vi "test-ElevatorSim-min-max.vi"() -> (3 "Test Passed":bool)   [LabVIEW 2019]
uses:
  <vilib>/Rock Robotics/WPI/ThirdParty/JAS_Junk/TrajLib/DCMOTOR.CTL
  <vilib>/Rock Robotics/WPI/ThirdParty/JAS_Junk/TrajLib/ELEVATOR_SIM.ctl
  <vilib>/Rock Robotics/WPI/ThirdParty/JAS_Junk/TrajLib/LINEAR_SYSTEM_SIM.ctl
  <vilib>/Rock Robotics/WPI/ThirdParty/JAS_Junk/TrajLib/LINEAR_SYSTEM.ctl
  <vilib>/Analysis/Matrix/Datatypes/RealMatrix.ctl
  <vilib>/Rock Robotics/WPI/ThirdParty/JAS_Junk/TrajLib/DCMotor_New.vi
  <vilib>/Rock Robotics/WPI/ThirdParty/JAS_Junk/TrajLib/Units_RotationsPerMinuteToRadiansPerSecond.vi
  <vilib>/Rock Robotics/WPI/ThirdParty/JAS_Junk/TrajLib/MatBuilder_Create.vi
  <vilib>/Rock Robotics/WPI/ThirdParty/JAS_Junk/TrajLib/MatBuilder_Fill.vi
  <vilib>/Rock Robotics/WPI/ThirdParty/JAS_Junk/TrajLib/MatrixHelper_Zero.vi
  <vilib>/Rock Robotics/WPI/ThirdParty/JAS_Junk/TrajLib/LinearSystem_New.vi
  <vilib>/Rock Robotics/WPI/ThirdParty/JAS_Junk/TrajLib/Trajectory_Library.lvlib
  <vilib>/Analysis/Matrix/NI_Matrix.lvlib
panel:
  in  "Tab Control":enum32{"Page 2", "Page 6", "Page 7"}(tab)
  out "Elevator Motor":T1 {"Jr_KgM2" format="%13.5p"; "L_H" format="%13.5p"; "Kt_NMPerAmp" format="%13.5p"; "KvINV_RadPerSecPerVolt" format="%13.5p"; "R_Ohms" format="%13.5p"; "FreeSpeed_RadPerSec" format="%13.5p"; "FreeCurrent_Amps" format="%13.5p"; "StallCurrent_Amps" format="%13.5p"; "StallTorque_NM" format="%13.5p"; "nominalVoltage_Volts" format="%13.5p"}
  out "Elevator Simulaation":T2 {"GearBox"."Jr_KgM2" format="%13.5p"; "GearBox"."L_H" format="%13.5p"; "GearBox"."Kt_NMPerAmp" format="%13.5p"; "GearBox"."KvINV_RadPerSecPerVolt" format="%13.5p"; "GearBox"."R_Ohms" format="%13.5p"; "GearBox"."FreeSpeed_RadPerSec" format="%13.5p"; "GearBox"."FreeCurrent_Amps" format="%13.5p"; "GearBox"."StallCurrent_Amps" format="%13.5p"; "GearBox"."StallTorque_NM" format="%13.5p"; "GearBox"."nominalVoltage_Volts" format="%13.5p"}
  out "Velocity":cluster{"Voltage":dbl}(graph)
  out "PV Chart":cluster{dbl}(graph)
  out "At Top":bool
  out "At Bottom":bool
  out "PV Chart 2":cluster{dbl}(graph)
  out "At Bottom 2":bool
  out "At Top 2":bool
  out "Velocity 2":cluster{"Voltage":dbl}(graph)
  # "<States, 1>"
  # "<Outputs, 1>"
  # "<Inputs, 1>"
  # "<Outputs, 1>"
  # "<States,States>"
  # "<States,Inputs>"
  # "<Outputs,States>"
  # "<Outputs,Inputs>"
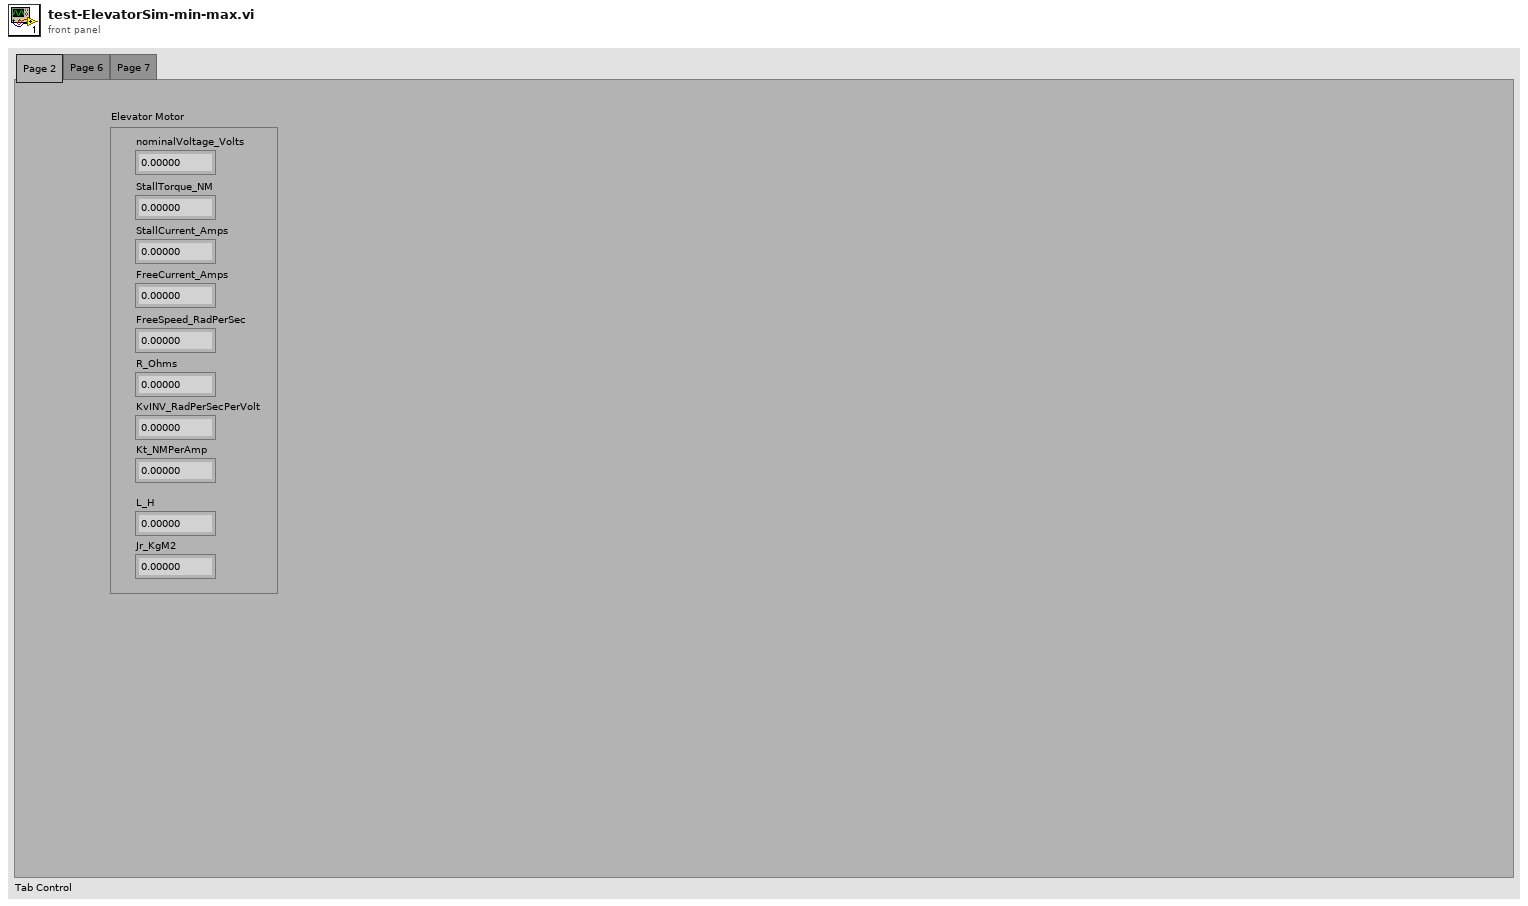
[diagram p1: front panel]
types:
  T1 = typedef "Trajectory_Library.lvlib/DCMOTOR.CTL" = cluster{"nominalVoltage_Volts":dbl, "StallTorque_NM":dbl, "StallCurrent_Amps":dbl, "FreeCurrent_Amps":dbl, "FreeSpeed_RadPerSec":dbl, "R_Ohms":dbl, "KvINV_RadPerSecPerVolt":dbl, "Kt_NMPerAmp":dbl, "L_H":dbl, "Jr_KgM2":dbl}
  T2 = typedef "Trajectory_Library.lvlib/ELEVATOR_SIM.ctl" = cluster{"LinearSystemSim":T3, "GearBox":T1, "Gearing":dbl, "DrumRadius_M":dbl, "MinHeight_M":dbl, "MaxHeight_M":dbl, "CarriageMass_Kg":dbl}
  T3 = typedef "Trajectory_Library.lvlib/LINEAR_SYSTEM_SIM.ctl" = cluster{"m_Plant":T4, "m_X":T5, "m_Y":T5, "m_U":T5, "MeasureStdDev":T5}
  T4 = typedef "Trajectory_Library.lvlib/LINEAR_SYSTEM.ctl" = cluster{"m_A":T5, "m_B":T5, "m_C":T5, "m_D":T5, "States":i32, "Inputs":i32, "Outputs":i32}
  T5 = typedef "NI_Matrix.lvlib/RealMatrix.ctl" = dbl[][]
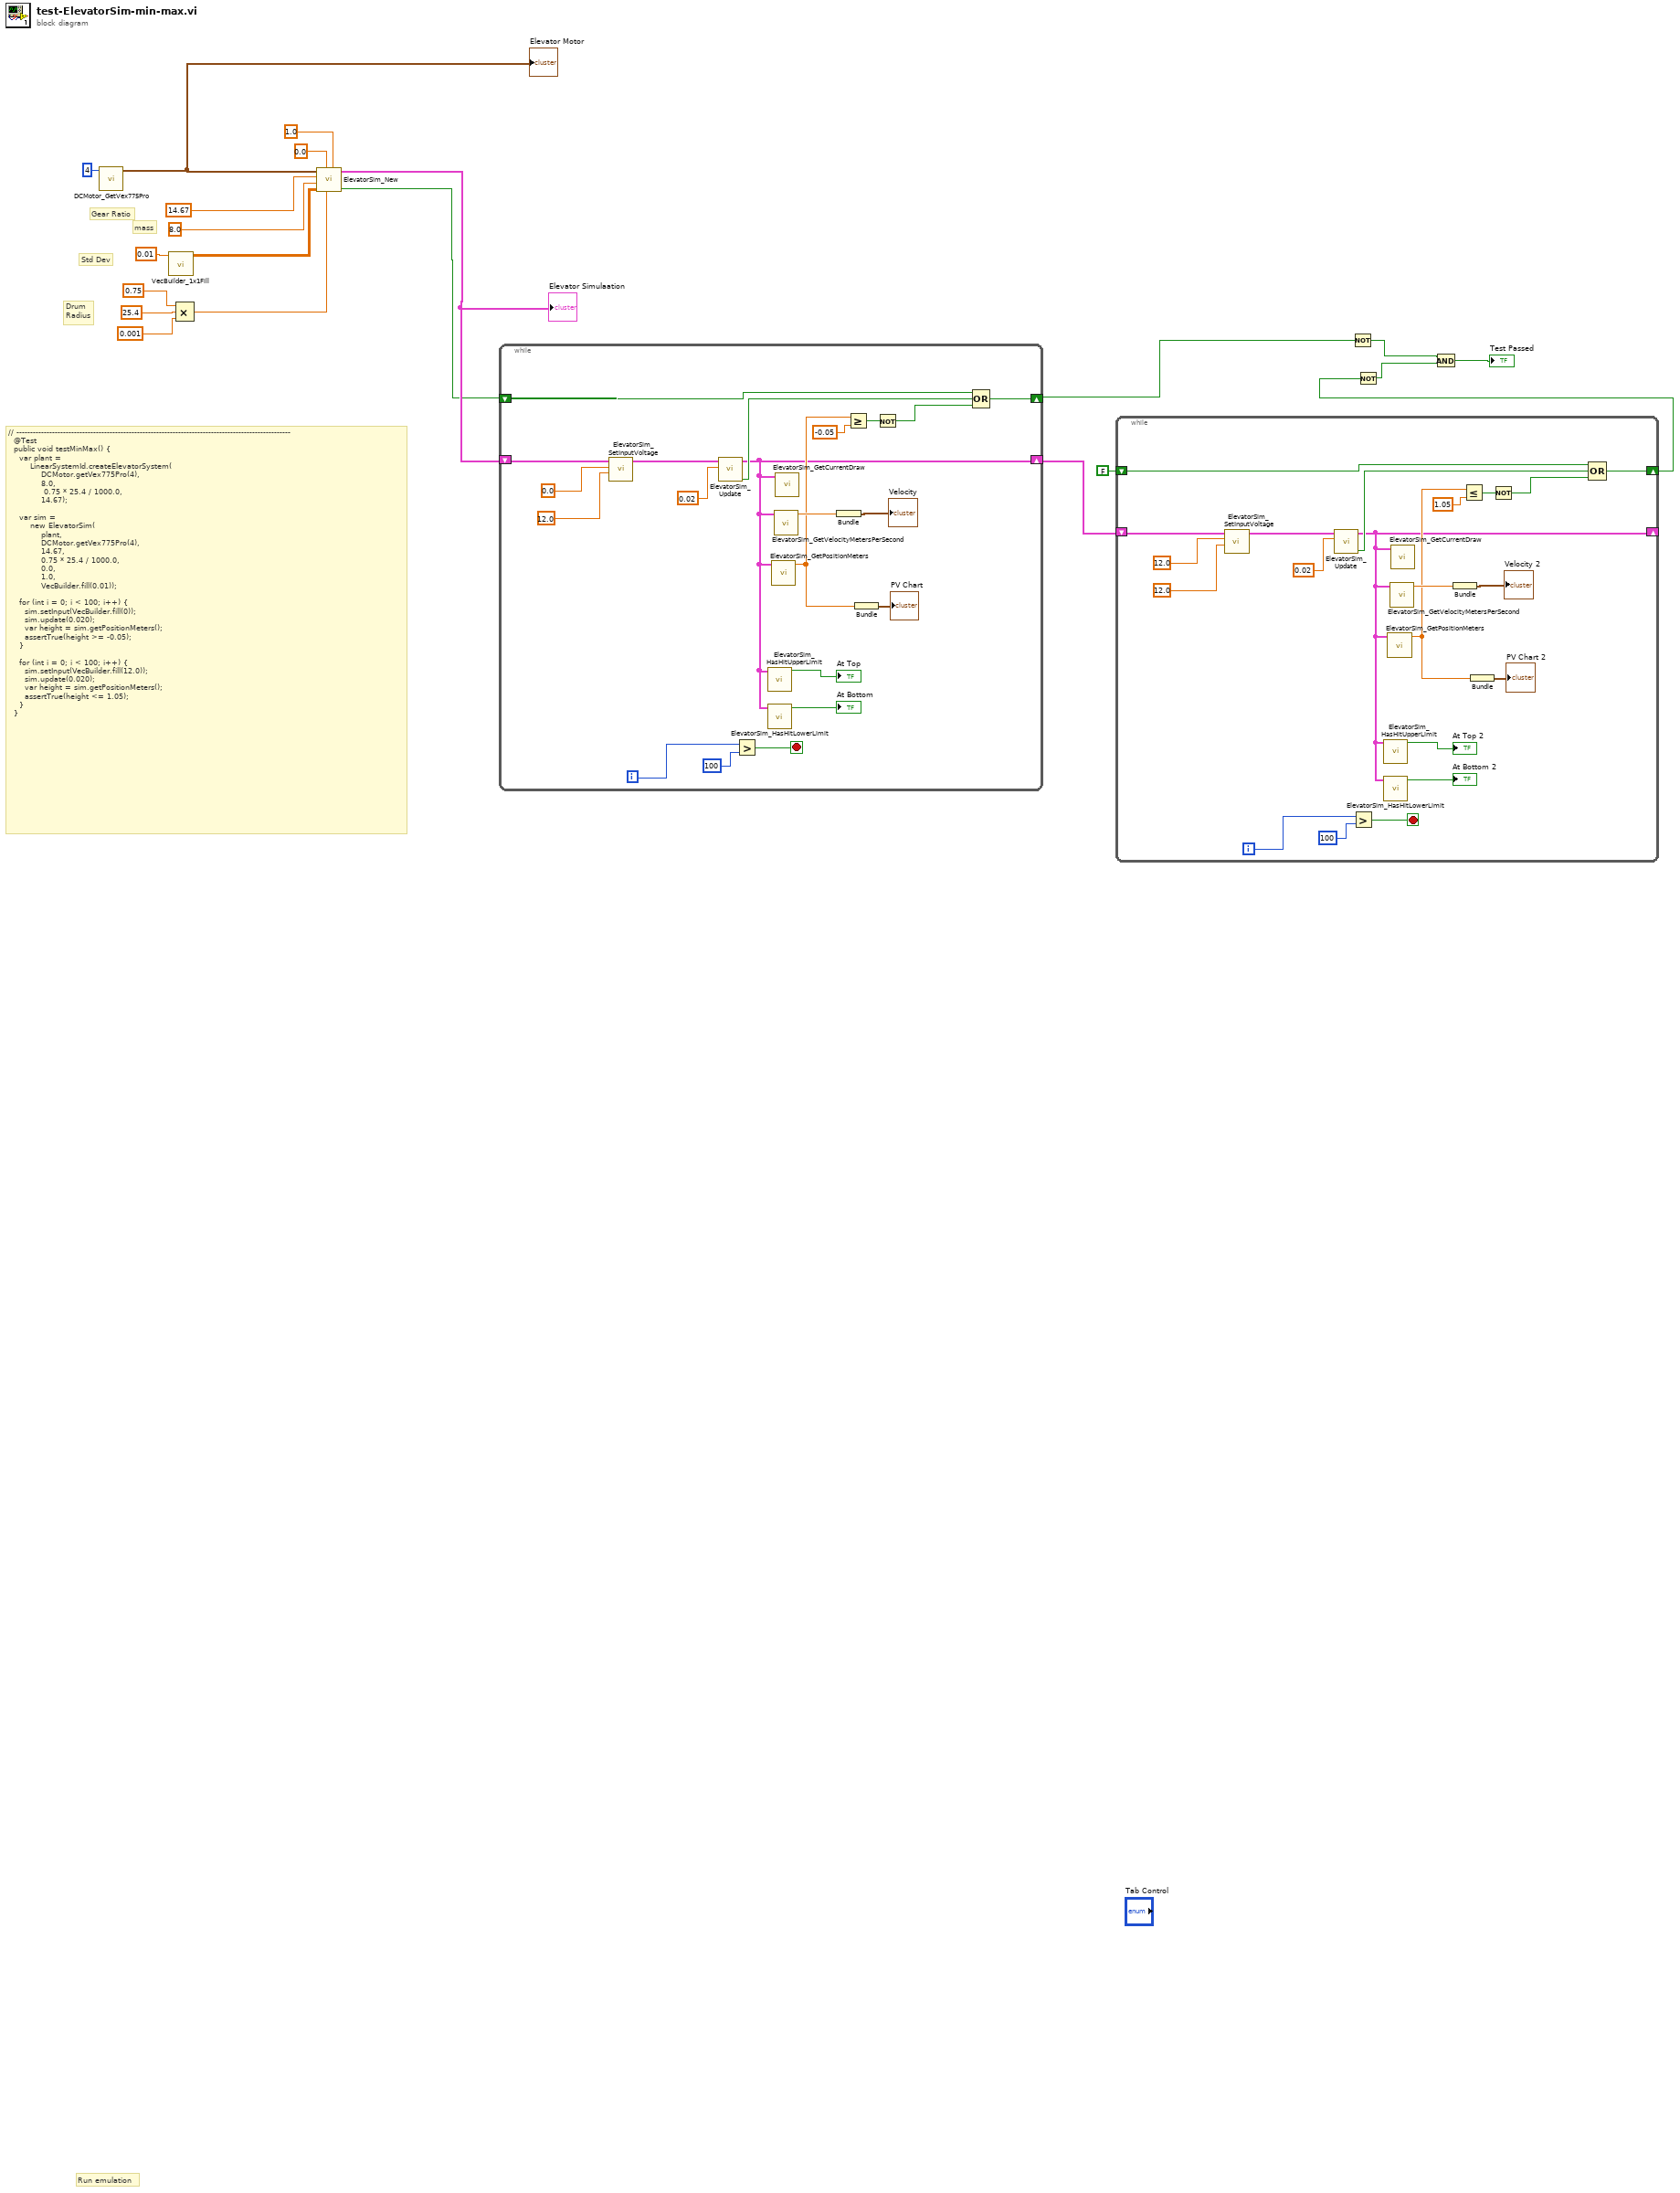
[diagram p0: block diagram]
diagram:
  # "Drum\nRadius"
  # "Std Dev"
  # "Gear Ratio"
  # "mass"
  # "// ----------------------------------------------------------------------------------------------------\n  @Test\n  public void testMinMax() {\n    var plant =\n        LinearSystemId.createElevatorSystem(\n            DCMotor.getVex775Pro(4), \n            8.0, \n             0.75 * 25.4 / 1000.0, \n            14.67);\n\n    var sim =\n        new ElevatorSim(\n            plant,\n            DCMotor.getVex775Pro(4),\n            14.67,\n            0.75 * 25.4 / 1000.0,\n            0.0,\n            1.0,\n            VecBuilder.fill(0.01));\n\n    for (int i = 0; i < 100; i++) {\n      sim.setInput(VecBuilder.fill(0));\n      sim.update(0.020);\n      var height = sim.getPositionMeters();\n      assertTrue(height >= -0.05);\n    }\n\n    for (int i = 0; i < 100; i++) {\n      sim.setInput(VecBuilder.fill(12.0));\n      sim.update(0.020);\n      var height = sim.getPositionMeters();\n      assertTrue(height <= 1.05);\n    }\n  }"
  # "Run emulation"
  n1 = call <vilib>:"DCMotor_GetVex775Pro.vi"("Num Motors"=4) -> ("DCMOTOR"=w6:T1)  [unwired: 10 in]
  "Elevator Motor" <- w6
  n2 = call <vilib>:"VecBuilder_1x1Fill.vi"("R0_C0"=0.01) -> ("output matrix"=w2:T5)  [unwired: 10 in]
  n3 = Compound Arithmetic op=MULTIPLY(0.75 ("value"), 25.4 ("value"), 0.001 ("value")) -> (w5:dbl)
  n4 = call <vilib>:"ElevatorSim_New.vi"("MaxHeight_Meters"=1.0, "DrumRadius_Meters"=w5, "MinHeight_Meters"=0.0, "MeasurementStdDev"=w2, "CarriageMass_Kg"=8.0 ("G"), "Gearing"=14.67, "GearBox"=w6) -> ("Error"=w1:bool, "ElevatorSim"=w7:T2)  [unwired: 3 in]
  "Elevator Simulaation" <- w7
  n5 = while {
    shift-right: [w24] -> w12
    shift-left: w7 -> [w31]
    shift-right: [w32] -> w18
    shift-left: w1 -> [w33]
    i -> [w37]
    stop <- w35 stop-if-true
    n6 = call <vilib>:"ElevatorSim_SetInputVoltage.vi"("Battery_Volts"=12.0, "Input_Voltage"=0.0, "in ElevatorSim"=w31) -> ("out ElevatorSim"=w30:T2)  [unwired: 8 in]
    n7 = call <vilib>:"ElevatorSim_Update.vi"("dT_Seconds"=0.02, "in ElevatorSim"=w30) -> ("Error"=w34:bool, "out ElevatorSim"=w24:T2)  [unwired: 8 in]
    n8 = Greater?(x=w37, y=100) -> (0:w35:bool)
    n9 = call <vilib>:"ElevatorSim_HasHitUpperLimit.vi"("ElevatorSim"=w24) -> ("At HIgh LImit"=→"At Top":bool)  [unwired: 10 in]
    n10 = call <vilib>:"ElevatorSim_HasHitLowerLimit.vi"("ElevatorSim"=w24) -> ("AtLowLimit"=→"At Bottom":bool)  [unwired: 10 in]
    n11 = call <vilib>:"ElevatorSim_GetPositionMeters.vi"("ElevatorSim"=w24) -> ("Position_Meters"=w27:dbl)  [unwired: 10 in]
    n12 = call <vilib>:"ElevatorSim_GetVelocityMetersPerSecond.vi"("ElevatorSim"=w24) -> ("Velocity_MetersPerSec"=w38:dbl)  [unwired: 10 in]
    n13 = call <vilib>:"ElevatorSim_GetCurrentDraw.vi"("ElevatorSim"=w24) -> ()  [unwired: 10 in, 1 out]
    n14 = Bundle("Velocity_MetersPerSec"=w38) -> (→"Velocity":cluster{"Velocity_MetersPerSec":dbl})  [unwired: 1 in]
    n15 = Greater Or Equal?(x=w27, y=-0.05) -> (x >= y?=w25:bool)
    n16 = Bundle("Position_Meters"=w27) -> (→"PV Chart":cluster{"Position_Meters":dbl})  [unwired: 1 in]
    n17 = Not(x=w25) -> (.not. x?=w23:bool)
    n18 = Compound Arithmetic op=OR(w33, w34, w23) -> (w32:bool)
  }
  n19 = while {
    shift-right: [w45] -> _
    shift-left: w12 -> [w52]
    shift-right: [w53] -> w11
    shift-left: FALSE -> [w54]
    i -> [w58]
    stop <- w56 stop-if-true
    n20 = call <vilib>:"ElevatorSim_SetInputVoltage.vi"("Battery_Volts"=12.0, "Input_Voltage"=12.0, "in ElevatorSim"=w52) -> ("out ElevatorSim"=w51:T2)  [unwired: 8 in]
    n21 = call <vilib>:"ElevatorSim_Update.vi"("dT_Seconds"=0.02, "in ElevatorSim"=w51) -> ("Error"=w55:bool, "out ElevatorSim"=w45:T2)  [unwired: 8 in]
    n22 = Greater?(x=w58, y=100) -> (0:w56:bool)
    n23 = call <vilib>:"ElevatorSim_HasHitUpperLimit.vi"("ElevatorSim"=w45) -> ("At HIgh LImit"=→"At Top 2":bool)  [unwired: 10 in]
    n24 = call <vilib>:"ElevatorSim_HasHitLowerLimit.vi"("ElevatorSim"=w45) -> ("AtLowLimit"=→"At Bottom 2":bool)  [unwired: 10 in]
    n25 = call <vilib>:"ElevatorSim_GetPositionMeters.vi"("ElevatorSim"=w45) -> ("Position_Meters"=w48:dbl)  [unwired: 10 in]
    n26 = call <vilib>:"ElevatorSim_GetVelocityMetersPerSecond.vi"("ElevatorSim"=w45) -> ("Velocity_MetersPerSec"=w59:dbl)  [unwired: 10 in]
    n27 = call <vilib>:"ElevatorSim_GetCurrentDraw.vi"("ElevatorSim"=w45) -> ()  [unwired: 10 in, 1 out]
    n28 = Bundle("Velocity_MetersPerSec"=w59) -> (→"Velocity 2":cluster{"Velocity_MetersPerSec":dbl})  [unwired: 1 in]
    n29 = Less Or Equal?(x=w48, y=1.05) -> (x <= y?=w46:bool)
    n30 = Bundle("Position_Meters"=w48) -> (→"PV Chart 2":cluster{"Position_Meters":dbl})  [unwired: 1 in]
    n31 = Not(x=w46) -> (.not. x?=w44:bool)
    n32 = Compound Arithmetic op=OR(w54, w55, w44) -> (w53:bool)
  }
  n33 = Not(x=w18) -> (.not. x?=w17:bool)
  n34 = Not(x=w11) -> (.not. x?=w10:bool)
  n35 = Compound Arithmetic op=AND(w17, w10) -> (→"Test Passed":bool)
